vi "ParseURL.vi"(11 "url":string) -> (1 "port":i32, 2 "base url":string, 3 "path":string)   [LabVIEW 2020]
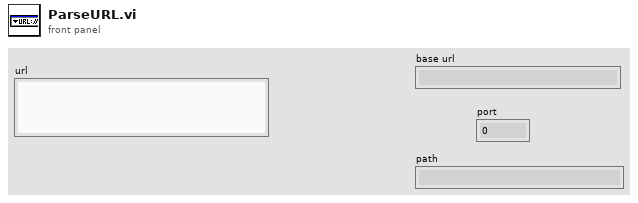
[diagram p1: front panel]
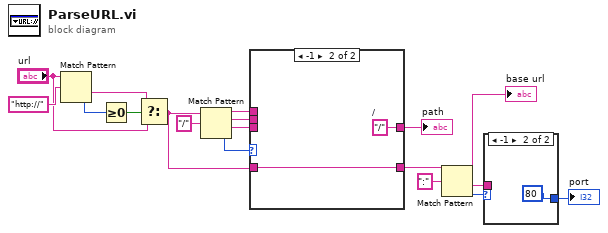
[diagram p0: block diagram]
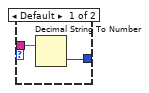
[diagram p2: hidden frame]
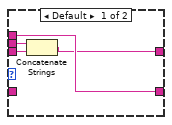
[diagram p3: hidden frame]
diagram:
  n1 = Match Pattern(string="url", regular expression="http://") -> (after substring=w14:string, offset past match=w16:i32)  [unwired: 1 in, 2 out]
  n2 = Greater Or Equal To 0?(x=w16) -> (x >= 0?=w15:bool)
  n3 = Select(t=w14, s=w15, f="url") -> (s? t:f=w9:string)
  n4 = Match Pattern(string=w9, regular expression="/") -> (before substring=w5:string, match substring=w1:string, after substring=w3:string, offset past match=w12:i32)  [unwired: 1 in]
  n5 = case shown="-1" w12 {
    tunnel: [w22 w24] -> w10
    tunnel: w9 -> [_ w24]
    tunnel: w5 -> [w22 _]
    tunnel: [w19 w23] -> w4
    tunnel: w3 -> [w20 _]
    tunnel: w1 -> [w21 _]
    frame Default {
      n6 = Concatenate Strings(w21, w20) -> (w19:string)
    }
    frame -1 {
      w23 = "/"  # /
    }
  }
  "path" <- w4
  n7 = Match Pattern(string=w10, regular expression=":") -> (before substring=→"base url":string, after substring=w6:string, offset past match=w8:i32)  [unwired: 1 in, 1 out]
  n8 = case shown="-1" w8 {
    tunnel: [w25 80] -> w7
    tunnel: w6 -> [w26 _]
    frame Default {
      n9 = Decimal String To Number(string=w26) -> (number=w25:i32)  [unwired: 2 in, 1 out]
    }
    frame -1 {
    }
  }
  "port" <- w7
